vi "VI Server Control N2 Act.vi"(0 "command text in":string[](array[string])) -> ()   [LabVIEW 2021]
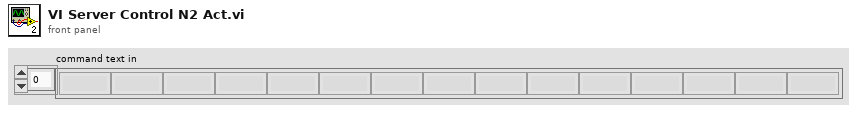
[diagram p1: front panel]
types:
  T1 = typedef "VI Server Control N2.ctl" = cluster{"VI name":string, "Control":string[], "Value":dbl[], "Boolean?":dbl[], "Wait Option":enum32{"Wait Until", "Do Not Wait"}, "wait (sec)":dbl, "Control to End":string, "finish boolean?":enum32{"boolean", "not boolean"}, "Condition":T2, "Target Value":dbl, "xxx%":dbl, "update every (s)":dbl, "Timeout (sec)":dbl}
  T2 = typedef "condition.ctl" = enum16{"within xxx% of target value", "<= target value", ">= target value", "= target value", "Boolean ON", "Boolean OFF"}
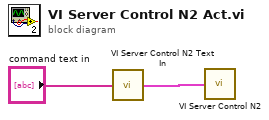
[diagram p0: block diagram]
diagram:
  n1 = call "VI Server Control N2 Text In.vi"("command text in"="command text in") -> ("VI Server Control N2"=w1:T1)
  n2 = call "VI Server Control N2.vi"("VI Server Control N2"=w1) -> ()
